vi "Get BLISS_Load and Save Default Server List.vi"(8 "error in (no error)":errorcluster) -> (0 "error out":errorcluster, 2 "Server Names (Dup)":string[](array[string]), 3 "File Ref Out":refnum<file>)   [LabVIEW 2020]
uses:
  MC5e Gobal_Variables.vi
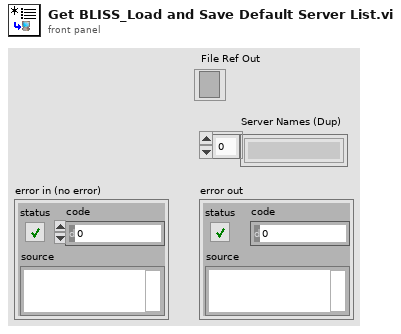
[diagram p1: front panel]
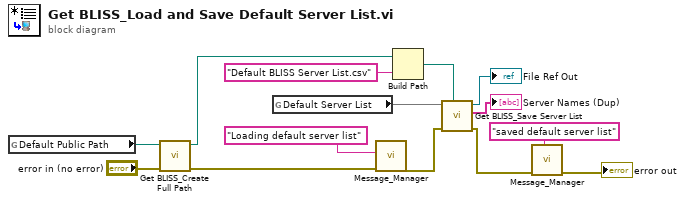
[diagram p0: block diagram]
diagram:
  n1 = global read "MC5e Gobal_Variables.vi" "Default Public Path"() -> (w4:path)
  n2 = call "Get BLISS_Create Full Path.vi"("error in"="error in (no error)", "Path to Create"=w4) -> ("error out"=w2:errorcluster, "Path Out"=w1:path)  [unwired: 7 in, 1 out]
  n3 = global read "MC5e Gobal_Variables.vi" "Default Server List"() -> (w10)
  n4 = call "Message_Manager.vi"("error in"=w2, "New Entry"="Loading default server list") -> ("error out"=w9:errorcluster)  [unwired: 4 in, 5 out]
  n5 = Build Path(base path=w1, name or relative path="Default BLISS Server List.csv") -> (appended path=w14:path)
  n6 = call "Get BLISS_Save Server List.vi"("file path (use dialog)"=w14, "error in (no error)"=w9, "Server Names"=w10) -> ("error out"=w7:errorcluster, "Server Names (Dup)"=→"Server Names (Dup)":string[], "File Ref Out"=→"File Ref Out":refnum<file>)  [unwired: 6 in]
  n7 = call "Message_Manager.vi"("error in"=w7, "New Entry"="saved default server list") -> ("error out"=→"error out":errorcluster)  [unwired: 4 in, 5 out]
